vi "Get Driver Version.vi"(8 "error in (no error)":errorcluster) -> (0 "error out":errorcluster, 2 "Library Version":u32 format="%x")   [LabVIEW 2019, in "D2XX-lv.lvlib"]
uses:
  D2XX-lv.lvlib
  D2XX_Functions_7.0/D2XX.lvlib
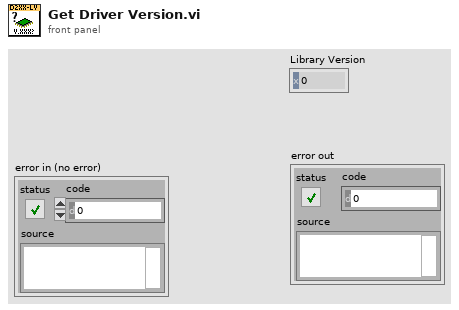
[diagram p1: front panel]
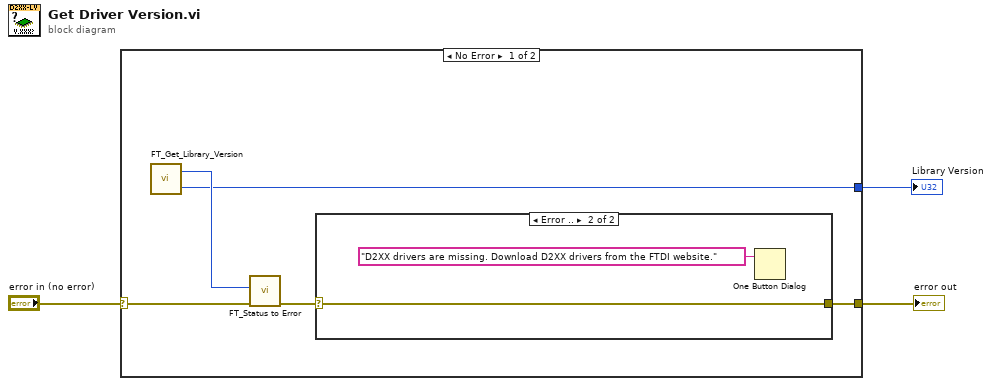
[diagram p0: block diagram]
diagram:
  n1 = case shown="No Error" "error in (no error)" {
    selector: "error in (no error)" -> [w8 w12]
    tunnel: [w4 w12] -> w2
    tunnel: [w6 _] -> w1
    frame No Error {
      n2 = call "FT_Get_Library_Version.vi"() -> ("Library Version"=w6:u32, "FT_Status"=w7:u32)
      n3 = call "FT_Status to Error.vi"("error in (no error)"=w8, "FT_Status"=w7) -> ("error out"=w5:errorcluster)  [unwired: 9 in]
      n4 = case shown="Error .." w5 {
        selector: w5 -> [w9 w10]
        tunnel: [w9 w10] -> w4
        frame No Error {
        }
        frame Error {
          n5 = One Button Dialog(message="D2XX drivers are missing. Download D2XX drivers from the FTDI website.") -> ()  [unwired: 1 in, 1 out]
        }
      }
    }
    frame Error {
    }
  }
  "error out" <- w2
  "Library Version" <- w1
